vi "Init Runtime.vi"(8 "error in (no error)":errorcluster, 10 "data allocations":T1, 11 "Update Tag Config in":refnum<class "Update Tag Config.lvclass">) -> (0 "error out":errorcluster, 2 "Skip":bool, 3 "Update Tag Config out":refnum<class "Update Tag Config.lvclass">)   [LabVIEW 2018, in "Update Tag Config.lvclass"]
uses:
  Update Tag Config.lvclass
  C:/Git/DCAF-Sequencer-Module/Prototype/classes/Step/Config/Step Config.lvclass
  <vilib>/NI/Tag Bus Module Framework/channel/data tables.ctl
  <vilib>/NI/Tag Bus/dictionary/data dictionary.lvclass
  <vilib>/NI/Tag Bus/dictionary table pair.ctl
  <vilib>/NI/Tag Bus/table/data table.ctl
  Execution/Update Tag.lvclass
  C:/Git/DCAF-Sequencer-Module/Prototype/classes/Step/Execution/Step.lvclass
  <vilib>/NI/Tag Bus Module Framework/channel/TBM channel.lvclass/TBM channel.ctl
  <vilib>/NI/Tag Bus/tag/tag descriptor.lvclass/tag descriptor.ctl
  <vilib>/NI/Tag Bus Module Framework/channel/TBM channel.lvclass
  C:/Program Files (x86)/National Instruments/LabVIEW 2018/vi.lib/NI/Tag Bus/tag/tag descriptor.lvclass
  <vilib>/NI/Tag Bus/dictionary/locate tag.vi
  <vilib>/NI/Tag Bus/tag/tag descriptor.lvclass
  <vilib>/NI/Tag Bus/table/data table.lvlib
  <vilib>/NI/Tag Bus/tag bus.lvlib
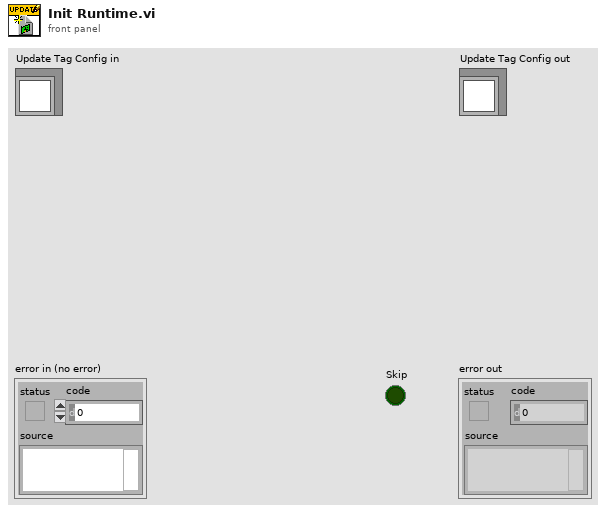
[diagram p1: front panel]
types:
  T1 = typedef "TBM channel.lvclass/data tables.ctl" = cluster{"input data":T2, "processing parameter":T2, "processing result":T2, "output data":T2}
  T2 = typedef "tag bus.lvlib/dictionary table pair.ctl" = cluster{"data dictionary":refnum<class "data dictionary.lvclass">, "data table":T3}
  T3 = typedef "tag bus.lvlib/data table.lvlib/data table.ctl" = cluster{"Double":dbl[], "Single":sgl[], "I64":i64[], "I32":i32[], "I16":i16[], "I8":i8[], "U64":u64[], "U32":u32[], "U16":u16[], "U8":u8[], "Boolean":bool[], "String":string[], "Array of Double":cluster{"DBL Array":dbl[]}[], "Array of Single":cluster{"SGL Array":sgl[]}[], "Array of I64":cluster{"I64 Array":i64[]}[], "Array of I32":cluster{"I32 Array":i32[]}[], "Array of I16":cluster{"I16 Array":i16[]}[], "Array of I8":cluster{"I8 Array":i8[]}[], "Array of U64":cluster{"U64 Array":u64[]}[], "Array of U32":cluster{"U32 Array":u32[]}[], "Array of U16":cluster{"U16 Array":u16[]}[], "Array of U8":cluster{"U8 Array":u8[]}[], "Array of Boolean":cluster{"Boolean Array":bool[]}[], "Array of String":cluster{"String Array":string[]}[]}
  T4 = typedef "tag bus.lvlib/tag descriptor.lvclass/Data Type.ctl" = enum16{"Double", "Single", "I64", "I32", "I16", "I8", "U64", "U32", "U16", "U8", "Boolean", "String", "Array of Double", "Array of Single", "Array of I64", "Array of I32", "Array of I16", "Array of I8", "Array of U64", "Array of U32", "Array of U16", "Array of U8", "Array of Boolean", "Array of String"}
  T5 = typedef "TBM channel.lvclass/channel classification.ctl" = enum16{"input data", "output data", "processing parameter", "processing result"}
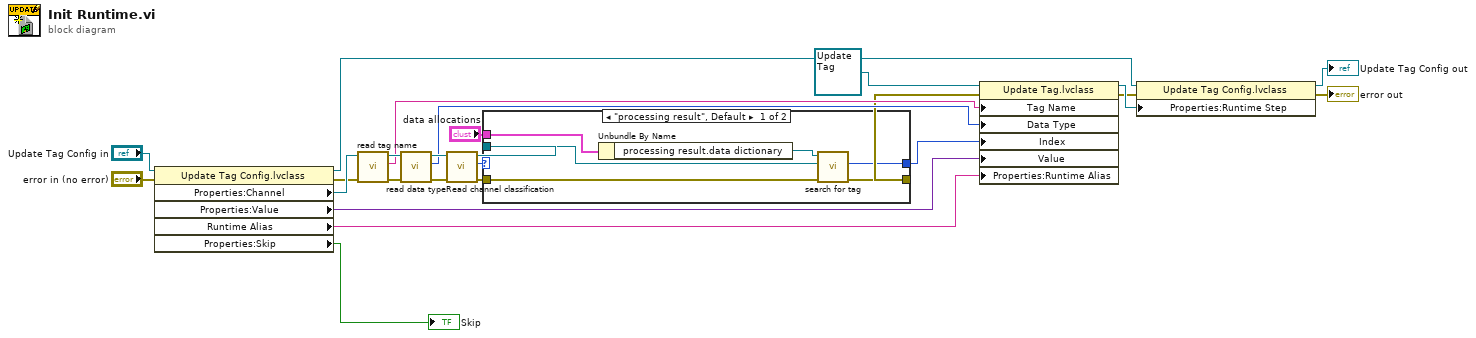
[diagram p0: block diagram]
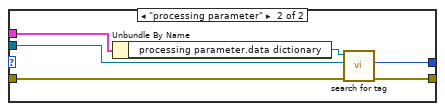
[diagram p2: hidden frame]
diagram:
  n1 = property class="Update Tag Config.lvclass"(reference="Update Tag Config in", error in="error in (no error)") -> (reference out=w24:refnum<class "Update Tag Config.lvclass">, error out=w9:errorcluster, "Properties:Channel"=w18:refnum<class "TBM channel.lvclass">, "Properties:Value"=w3:variant, "Runtime Alias"=w1:string, "Properties:Skip"=→"Skip":bool)
  n2 = call <vilib>:"read tag name.vi"("error in"=w9, "system tag in"=w18) -> ("error out"=w8:errorcluster, "name"=w15:string, "system tag out"=w17:refnum<class "TBM channel.lvclass">)  [unwired: 7 in]
  n3 = call <vilib>:"read data type.vi"("error in"=w8, "system tag in"=w17) -> ("error out"=w7:errorcluster, "data type"=w14:T4, "system tag out"=w16:refnum<class "TBM channel.lvclass">)  [unwired: 7 in]
  n4 = call <vilib>:"Read channel classification.vi"("error in"=w7, "channel in"=w16) -> ("error out"=w6:errorcluster, "channel classification"=w13:T5, "channel out"=w11:refnum<class "TBM channel.lvclass">)  [unwired: 7 in]
  n5 = case shown="\"processing result\", Default" w13 {
    tunnel: "data allocations" -> [w30 w37]
    tunnel: w11 -> [w26 w35]
    tunnel: [w29 w34] -> w10
    tunnel: w6 -> [w28 w33]
    tunnel: [w27 w32] -> w5
    frame "processing result", Default {
      n6 = Unbundle By Name(w30) -> ("processing result.data dictionary"=w31:refnum<class "data dictionary.lvclass">)
      n7 = call <vilib>:"search for tag.vi"("error in"=w28, "system tag"=w26, "data dictionary in"=w31) -> ("error out"=w27:errorcluster, "index"=w29:i32)  [unwired: 6 in, 1 out]
    }
    frame "processing parameter" {
      n8 = Unbundle By Name(w37) -> ("processing parameter.data dictionary"=w36:refnum<class "data dictionary.lvclass">)
      n9 = call <vilib>:"search for tag.vi"("error in"=w33, "system tag"=w35, "data dictionary in"=w36) -> ("error out"=w32:errorcluster, "index"=w34:i32)  [unwired: 6 in, 1 out]
    }
  }
  n10 = property class="Update Tag.lvclass"(reference=refnum<class "Update Tag.lvclass"> refnum ("Update Tag.lvclass"), error in=w5, "Tag Name"=w15, "Data Type"=w14, "Index"=w10, "Value"=w3, "Properties:Runtime Alias"=w1) -> (reference out=w22:refnum<class "Update Tag.lvclass">, error out=w21:errorcluster)
  n11 = property class="Update Tag Config.lvclass"(reference=w24, error in=w21, "Properties:Runtime Step"=w22) -> (reference out=→"Update Tag Config out":refnum<class "Update Tag Config.lvclass">, error out=→"error out":errorcluster)
